vi "9613 Empty Section Name--error.vi"(8 "error in":errorcluster) -> (0 "error out":errorcluster)   [LabVIEW 2024, in "Electronic Datasheet.lvlib"]
uses:
  Electronic Datasheet.lvlib
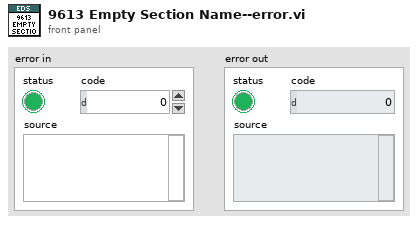
[diagram p1: front panel]
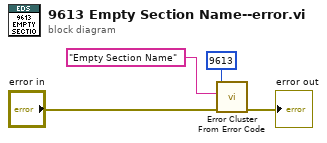
[diagram p0: block diagram]
diagram:
  n1 = call <vilib>:"Error Cluster From Error Code.vi"("error in (no error)"="error in", "error message (\"\")"="Empty Section Name" ("error message (\"\")"), "error code (0)"=9613) -> ("error out"=→"error out":errorcluster)  [unwired: 6 in]
